vi "Retrieve_memory_4Gb.vi"(9 "MB LIBRE OK":i64, 11 "MB MIN MEMORIA LIBRE":i64) -> ()   [LabVIEW 2015]
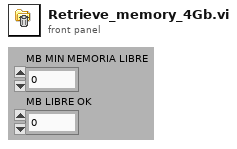
[diagram p1: front panel]
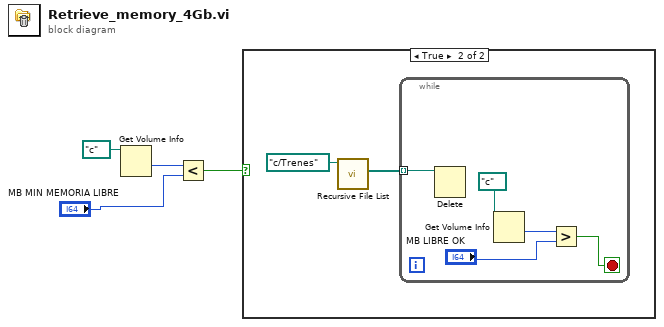
[diagram p0: block diagram]
diagram:
  n1 = Get Volume Info(11:path "c:/" ("path")) -> (1:w3:i64)  [unwired: 1 in, 5 out]
  n2 = Less?(x=w3, y="MB MIN MEMORIA LIBRE") -> (x < y?=w2:bool)
  n3 = case shown="True" w2 {
    frame False {
    }
    frame True {
      n4 = call <vilib>:"Recursive File List.vi"("Folder Path"=path "c:/Trenes") -> ("All Files in Dir"=w5:path[])  [unwired: 6 in, 4 out]
      n5 = while {
        tunnel: w5 -> [w11] mode=indexing
        stop <- w8 stop-if-true
        n6 = Delete(path (use dialog)=w11) -> ()  [unwired: 4 in, 3 out]
        n7 = Get Volume Info(11:path "c:/" ("path")) -> (1:w9:i64)  [unwired: 1 in, 5 out]
        n8 = Greater?(x=w9, y="MB LIBRE OK") -> (0:w8:bool)
      }
    }
  }
